vi "Register.vi"(8 "error in":errorcluster, 10 "TPCANHandle":T1 items=["PCAN_NONEBUS"=0, "PCAN_USBBUS1"=81, "PCAN_USBBUS2"=82, "PCAN_USBBUS3"=83, "PCAN_USBBUS4"=84, "PCAN_USBBUS5"=85, "PCAN_USBBUS6"=86, "PCAN_USBBUS7"=87, "PCAN_USBBUS8"=88, "PCAN_USBBUS9"=1289, "PCAN_USBBUS10"=1290, "PCAN_USBBUS11"=1291, "PCAN_USBBUS12"=1292, "PCAN_USBBUS13"=1293, "PCAN_USBBUS14"=1294, "PCAN_USBBUS15"=1295, "PCAN_USBBUS16"=1296], 11 "Message Waiter in":refnum<class "Message Waiter.lvclass">) -> (0 "error out":errorcluster, 3 "Message Waiter out":refnum<class "Message Waiter.lvclass">)   [LabVIEW 2018, in "PCANBasic.lvlib" / "Message Waiter.lvclass"]
uses:
  Message Waiter.lvclass
  TPCANHandle.ctl
  PCANBasic.lvlib
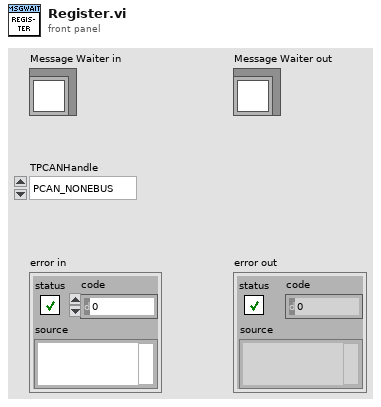
[diagram p1: front panel]
types:
  T1 = typedef "PCANBasic.lvlib/TPCANHandle.ctl" = u16
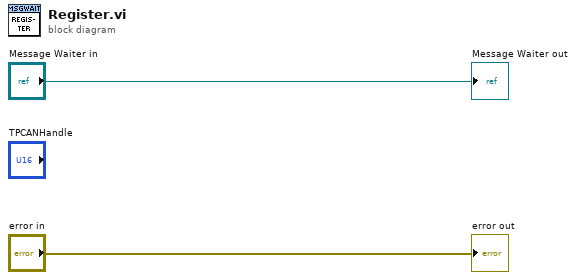
[diagram p0: block diagram]
diagram:
  "error out" <- "error in"
  "Message Waiter out" <- "Message Waiter in"
